vi "DC Hall.vi"(8 "error in":errorcluster) -> (0 "error out":errorcluster)   [LabVIEW 2025]
panel:
  in  "Temperature  channel":string="LakeShore 336 (12) A"
  in  "Save sweep":bool
  out "Slope":dbl format="%#_6p"
  out "T":dbl
  in  "Save file":path
  in  "Reset":bool
  in  "Master start":i64=2698
  in  "Save log":bool
  in  "Next":bool=TRUE
  out "End Index out":i32=-1
  in  "Start":i64
  in  "Monitor channel":string="LakeShore 336 (12) B Raw"
  in  "Signal channel":string="LakeShore 370 (13) R"
  in  "Status channel":string="B status"
  in  "Field channel":string="B"
  in  "Master labeling channel":string="T"
  in  "File Path":path=path "C:/Data/October_2025/102525/m003_111527_102525.tdms"
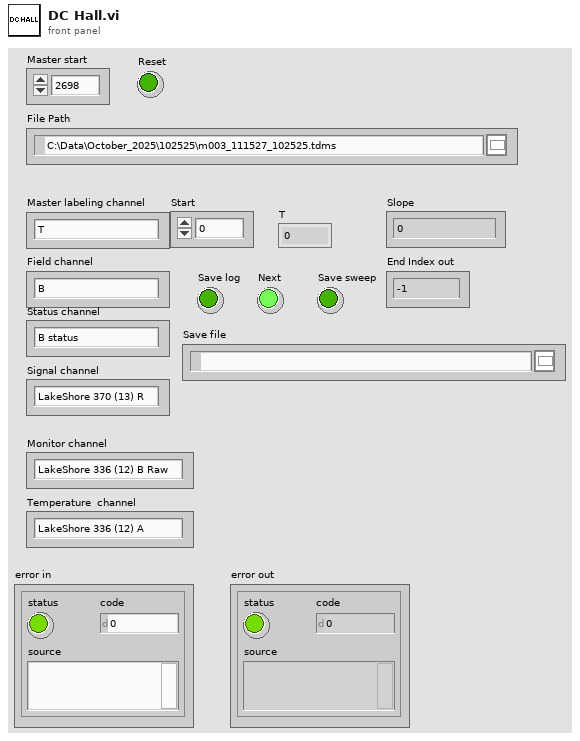
[diagram p1: front panel]
types:
  T1 = enum16{"open", "open or create", "create or replace", "create", "open (read-only)"}
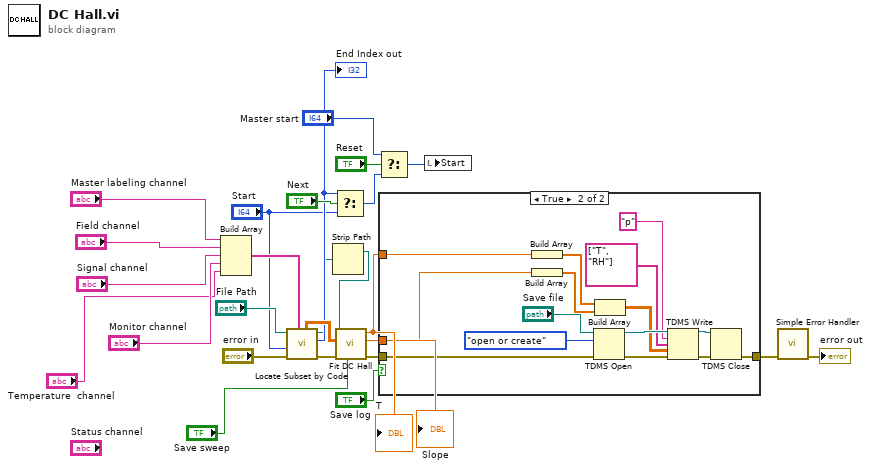
[diagram p0: block diagram]
diagram:
  n1 = Build Array("Master labeling channel", "Field channel", "Signal channel", "Monitor channel", "Temperature  channel") -> (w22:string[])
  n2 = call "Locate Subset by Code.vi"("Read channels"=w22, "error in"="error in", "Start"="Start", "File Path"="File Path") -> ("error out"=w17:errorcluster, "End Index out"=w15:i32, "file path out"=w4:path, "Data out"=w18:dbl[][])  [unwired: 2 in, 2 out]
  "End Index out" <- w15
  n3 = Strip Path(path=w4) -> (stripped path=w3:path)  [unwired: 1 out]
  n4 = Select(t=w15, s="Next", f="Start") -> (s? t:f=w12:i64)
  n5 = call "Fit DC Hall.vi"("Save?"="Save sweep", "error in"=w17, "Data"=w18, "Data folder"=w3) -> ("error out"=w8:errorcluster, "Slope"=w5:dbl, "T"=w6:dbl)  [unwired: 5 in]
  "T" <- w6
  "Slope" <- w5
  n6 = Select(t="Master start", s="Reset", f=w12) -> (s? t:f=w11:i64)
  n7 = case shown="True" "Save log" {
    tunnel: w8 -> [w27 w40]
    tunnel: [w27 w33] -> w7
    tunnel: w6 -> [_ w32]
    tunnel: w5 -> [_ w31]
    frame False {
    }
    frame True {
      n8 = Build Array(w32) -> (w30:dbl[])
      n9 = Build Array(w31) -> (w29:dbl[])
      n10 = TDMS Open(8:w40, 10:T1."open or create" ("operation (0:open)"), 11:"Save file") -> (0:w38:errorcluster, 3:w39:refnum<k34>)  [unwired: 4 in]
      n11 = Build Array(w30, w29) -> (w28:dbl[][])
      n12 = TDMS Write(0:w39, 5:"p" ("group name in (Untitled)"), 7:string[] ["T", "RH"] ("channel name(s) in (Untitled)"), 9:w28, 11:w38) -> (4:w34:refnum<k34>, 15:w35:errorcluster)  [unwired: 1 in, 2 out]
      n13 = TDMS Close(8:w35, 11:w34) -> (0:w33:errorcluster)  [unwired: 1 out]
    }
  }
  n14 = local write "Start"(w11) -> ()
  n15 = call <vilib>:"Simple Error Handler.vi"("error in (no error)"=w7) -> ("error out"=→"error out":errorcluster)  [unwired: 4 in, 4 out]
